vi "Read Core.vi"(8 "error in (no error)":errorcluster, 9 "Timeout (1s)":dbl[unit]=1.0, 11 "PVConnection in":refnum<class "SVConnection.lvclass">) -> (0 "error out":errorcluster, 1 "timed out":bool, 2 "PV":refnum<class "PV.lvclass">, 3 "PVConnection out":refnum<class "SVConnection.lvclass">)   [LabVIEW 2016, in "CS++SharedVariables.lvlib" / "SVConnection.lvclass"]
doc: "Read a process variable."
uses:
  SVConnection.lvclass
  C:/User/Brand/LVP/CSPP/Packages/CSPP_Core/Classes/CS++ProcessVariables/PVConnection/PVConnection.lvclass
  C:/User/Brand/LVP/CSPP/Packages/CSPP_Core/Classes/CS++BaseClasses/Base/CS++Base.lvclass
  ProcessVariable/PV.lvclass
  SVConnection.lvclass/SVConnection.ctl
  PVConnection/PVConnection.lvclass/PVConnection.ctl
  ProcessVariable/PV.lvclass/PV.ctl
  CS++BaseClasses/Base/CS++Base.lvclass/CS++Base.ctl
  ProcessVariable/Write Data.vi
  ProcessVariable/Write Error.vi
  ProcessVariable/Write Timestamp.vi
  ProcessVariable/Write status.vi
  ProcessVariable/Write Quality.vi
  PVConnection/PVConnection.lvclass
  Libraries/Utilities/CS++Utilities.lvlib
  CS++BaseClasses/Base/CS++Base.lvclass
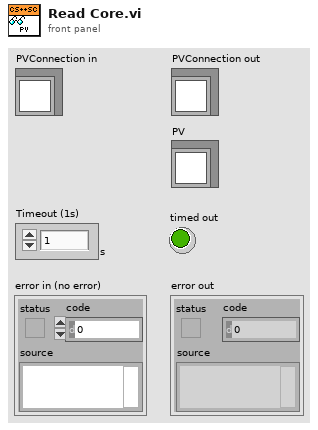
[diagram p1: front panel]
types:
  T1 = cluster{"Read Access":enum8{"Allowed", "Required", "None"}, "Write Access":enum8{"Allowed", "Required", "None"}}
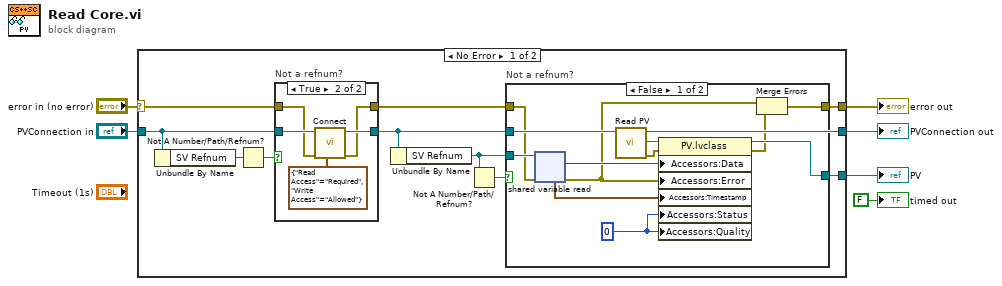
[diagram p0: block diagram]
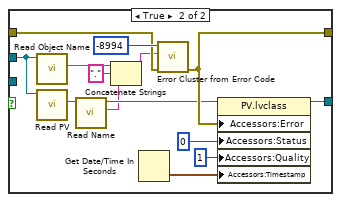
[diagram p3: hidden frame]
diagram:
  n1 = case shown="No Error" "error in (no error)" {
    selector: "error in (no error)" -> [w8 w50]
    tunnel: [w16 w50] -> w3
    tunnel: [w9 w51] -> w4
    tunnel: "PVConnection in" -> [w10 w51]
    tunnel: [w13 _] -> w2
    frame No Error {
      n2 = Unbundle By Name(w10) -> ("SV Refnum"=w12:refnum<k21>)
      n3 = Not A Number/Path/Refnum?(number/path/refnum=w12) -> (NaN/Path/Refnum?=w11:bool)
      n4 = case "Not a refnum?" shown="True" w11 {
        tunnel: w10 -> [w17 w23]
        tunnel: [w17 w22] -> w9
        tunnel: w8 -> [w18 w21]
        tunnel: [w18 w20] -> w7
        frame False {
        }
        frame True {
          n5 = call "Connect.vi"("Access (R/W allowed)"=T1 {"Read Access"=enum."Required", "Write Access"=enum."Allowed"}, "Error In"=w21, "PVConnection in"=w23) -> ("Error Out"=w20:errorcluster, "PVConnection out"=w22:refnum<class "SVConnection.lvclass">)  [unwired: 7 in]
        }
      }
      n6 = Unbundle By Name(w9) -> ("SV Refnum"=w14:refnum<k21>)
      n7 = Not A Number/Path/Refnum?(number/path/refnum=w14) -> (NaN/Path/Refnum?=w15:bool)
      n8 = case "Not a refnum?" shown="False" w15 {
        tunnel: w14 -> [w35 _]
        tunnel: w7 -> [w34 w48]
        tunnel: [w25 w46] -> w16
        tunnel: w9 -> [w33 w40]
        tunnel: [w29 w47] -> w13
        frame False {
          w30 = u32 0 ("status")
          n9 = shared-variable-read(w35, w34) -> (w24:errorcluster, w32:variant, w31:timestamp)  [unwired: 1 out]
          n10 = call "Read PV.vi"("PVConnection in"=w33) -> ("error out"=w27:errorcluster, "PV"=w28:refnum<class "PV.lvclass">)  [unwired: 8 in, 1 out]
          n11 = property class="PV.lvclass"(reference=w28, error in=w27, "Accessors:Data"=w32, "Accessors:Error"=w24, "Accessors:Timestamp"=w31, "Accessors:Status"=w30, "Accessors:Quality"=w30) -> (reference out=w29:refnum<class "PV.lvclass">, error out=w26:errorcluster)
          n12 = Merge Errors(w24, w26) -> (w25:errorcluster)
        }
        frame True {
          n13 = call "Read Object Name.vi"("Base in"=w40) -> ("Object Name"=w39:string)  [unwired: 8 in, 2 out]
          n14 = call "Read PV.vi"("PVConnection in"=w40) -> ("PV"=w42:refnum<class "PV.lvclass">)  [unwired: 8 in, 2 out]
          n15 = call "Read Name.vi"("PV in"=w42) -> ("Name"=w37:string, "PV out"=w41:refnum<class "PV.lvclass">)  [unwired: 8 in, 1 out]
          n16 = Concatenate Strings(w39, "." ("string"), w37) -> (w36:string)
          n17 = Get Date/Time In Seconds() -> (seconds since 1Jan1904=w43:timestamp)
          n18 = call "Error Cluster from Error Code.vi"("Error In"=w48, "Error Message (\"\")"=w36, "Error Code (0)"=-8994 ("error code (0)")) -> ("Error Out"=w46:errorcluster)  [unwired: 8 in]
          n19 = property class="PV.lvclass"(reference=w41, "Accessors:Error"=w46, "Accessors:Status"=u32 0 ("status"), "Accessors:Quality"=u64 1 ("quality"), "Accessors:Timestamp"=w43) -> (reference out=w47:refnum<class "PV.lvclass">)  [unwired: 1 in, 1 out]
        }
      }
    }
    frame Error {
    }
  }
  "error out" <- w3
  "PVConnection out" <- w4
  "PV" <- w2
  "timed out" <- FALSE ("timed out")
